vi "SubVI PhaseSpace.vi"() -> ()   [LabVIEW 2021]
uses:
  ctrOWLMarker.ctl
  ctlSeqFNs_SubVI PhaseSpace.ctl
  ctlPkgPhaseSpace.ctl
  ctlSeqFNs_SubVI ATI.ctl
  ctlTrialState.ctl
  ctlSeqFNs.ctl
  ctrSetsFlags.ctl
  ctrCommonFlags.ctl
  ctldistance2plane.ctl
  ctlRecording.ctl
  GLOBAL -MAIN.vi
  C:/Program Files/Phasespace/libowlsock.dll
panel:
  out "bias frame [R T]":dbl[][](array[numeric]) format="%#.2f"
  out "marker condition":bool[](array[boolean])
  in  "marker count":i32=14
  out "Hz":dbl(graph)
  out "save file":path
  in  "Read Cycle Time (s)":dbl=0.02 min=0.01 max=10.0 step=0.01 format="%.2f"
  out "recording?":bool
  out "markers obtained (err: <0)":u16
  out "markers":T1[](array[typedef])
  out "connected?":bool
  in  "server IP":string="192.168.1.230"
  in  "STOP":bool
  # "Parallel SubVI PhaseSpace"
  # "Acquires PhaseSpace data and Trigger signal\nSaves TDMS file."
  # "00   01  02  03   04  05   06  07  08  09   10  11   12  13"
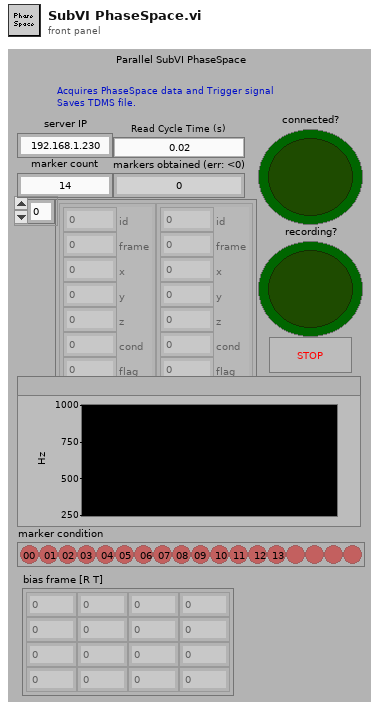
[diagram p1: front panel]
types:
  T1 = typedef "ctrOWLMarker.ctl" = cluster{"id":i32, "frame":i32, "x":sgl, "y":sgl, "z":sgl, "cond":sgl, "flag":u32}
  T2 = typedef "ctlPkgPhaseSpace.ctl" = cluster{"VIRef":refnum<vi>, "PhaseSpace":refnum<k34>, "PhaseSpace Ch names":string[], "Markers":T1[], "Markers Ch count":i32, "tick ini":i64, "ATI":refnum<queue>, "Trigger events":T3, "connected to server?":bool, "recording?":bool, "MAIN":refnum<queue>, "tick pre":i64, "Markers count":u16, "Data":dbl[][]}
  T3 = typedef "ctlTrialState.ctl" = enum16{"no events", "ready", "start", "hold", "stop", "end"}
  T4 = typedef "ctlSeqFNs_SubVI PhaseSpace.ctl" = enum16{"INITIALIZE", "IDLE", "BIAS", "READY", "SEND2MAIN", "LOG2TDMS", "TRIGGER", "END", "ERROR", "EXIT"}
  T5 = typedef "ctlSeqFNs.ctl" = enum16{"INITIALIZE MAIN", "UpdateProtocol", "UpdateBlockInfo", "UpdatePath", "INITIALIZE Sub", "IDLE", "Bias", "Ready", "RepeatTrial", "Events", "Get PS bias", "Get PhaseSpace", "Get ATI", "Finish", "End PhaseSpace", "End ATI", "ERROR", "EXIT"}
  T6 = typedef "ctlSeqFNs_SubVI ATI.ctl" = enum16{"INITIALIZE", "SET HANDLE", "IDLE", "READY", "SEND2MAIN", "CALIB Load", "BIAS", "TRIGGER", "END", "ERROR", "EXIT"}
  T7 = enum16{"ALIGN -CENTER", "ALIGN -TOP LEFT", "ALIGN -AS IS", "ALIGN -CUSTOM"}
  T8 = typedef "ctldistance2plane.ctl" = cluster{"frame":dbl[][]}
  T9 = typedef "ctlRecording.ctl" = cluster{"recording?":bool, "tdms file":refnum<k34>}
  T10 = typedef "ctrCommonFlags.ctl" = u16
  T11 = typedef "ctrSetsFlags.ctl" = u16
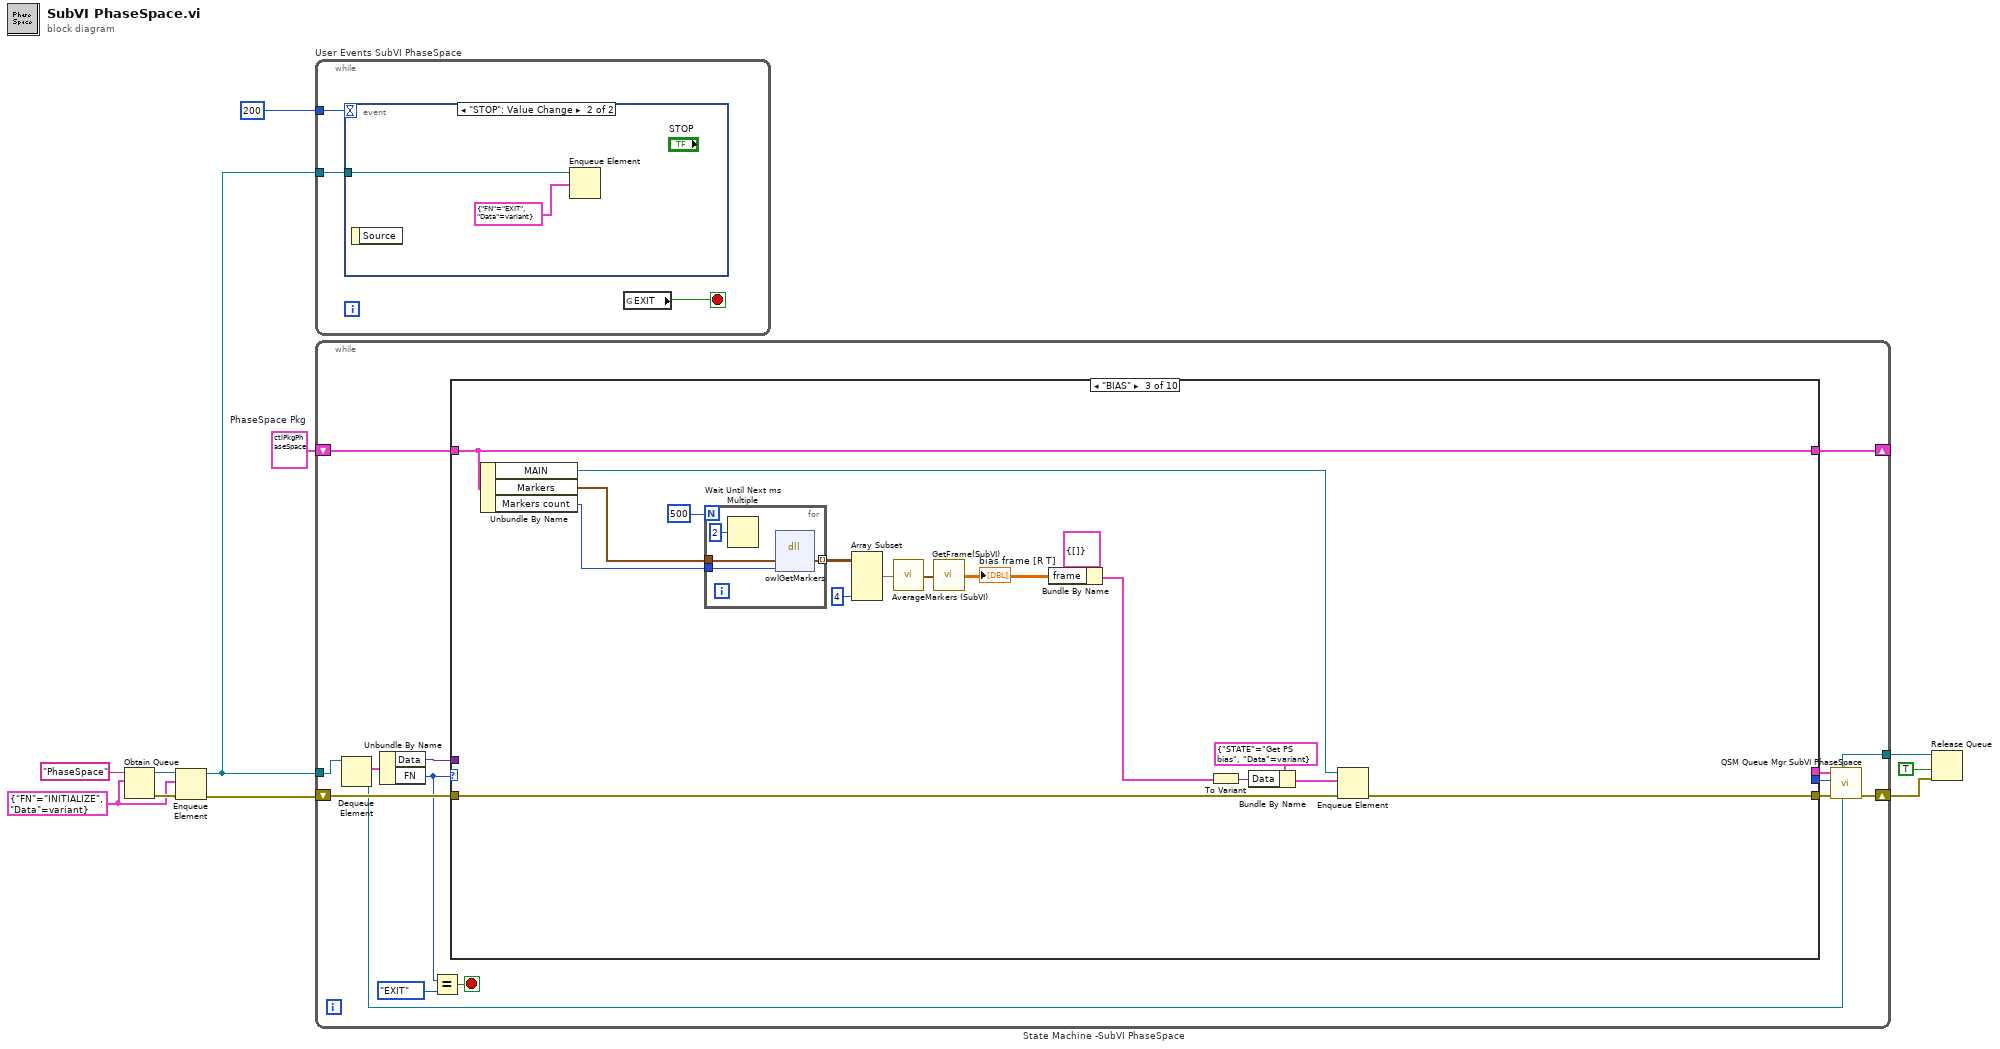
[diagram p0: block diagram]
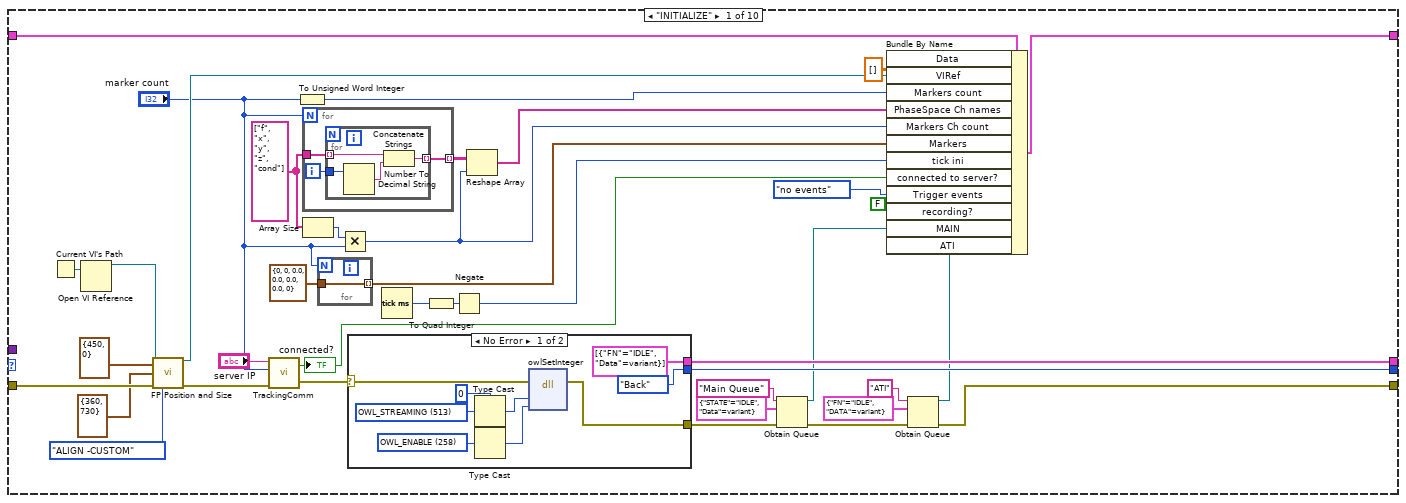
[diagram p2: hidden frame]
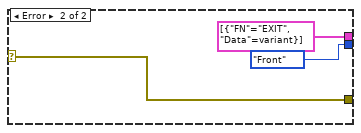
[diagram p3: hidden frame]
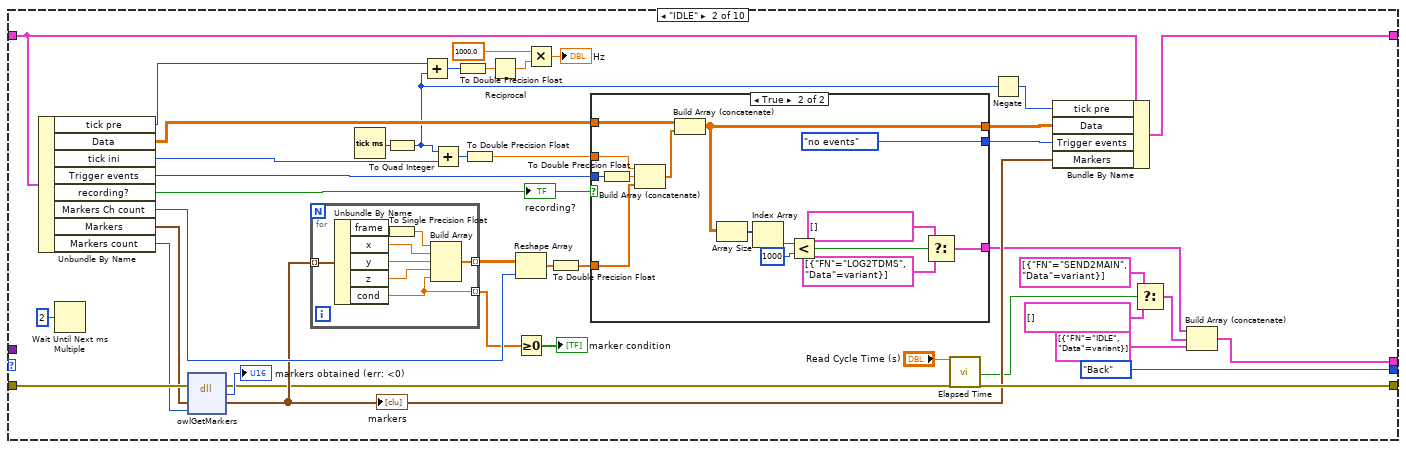
[diagram p4: hidden frame]
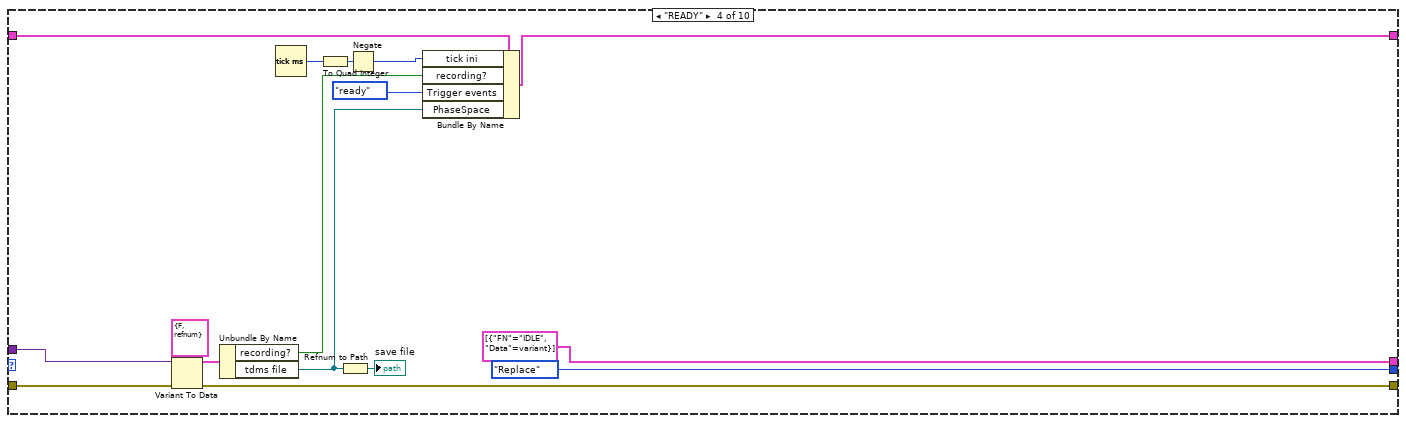
[diagram p6: hidden frame]
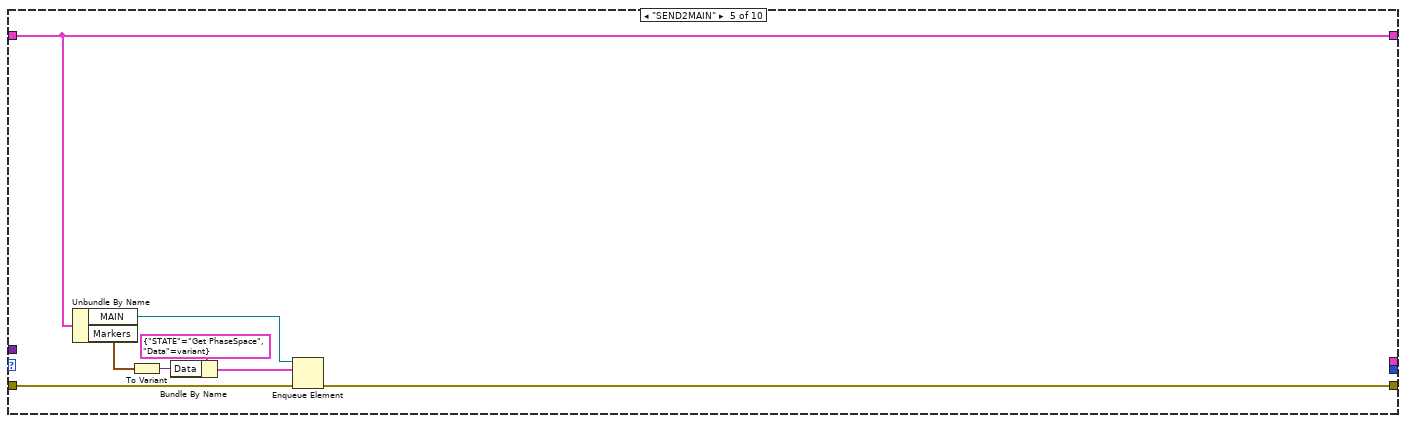
[diagram p7: hidden frame]
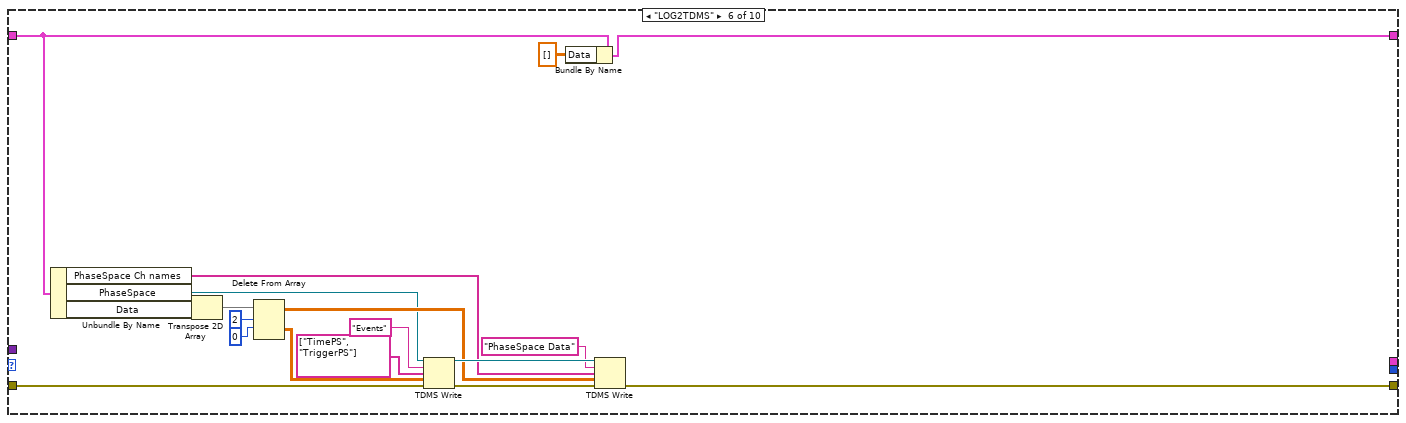
[diagram p8: hidden frame]
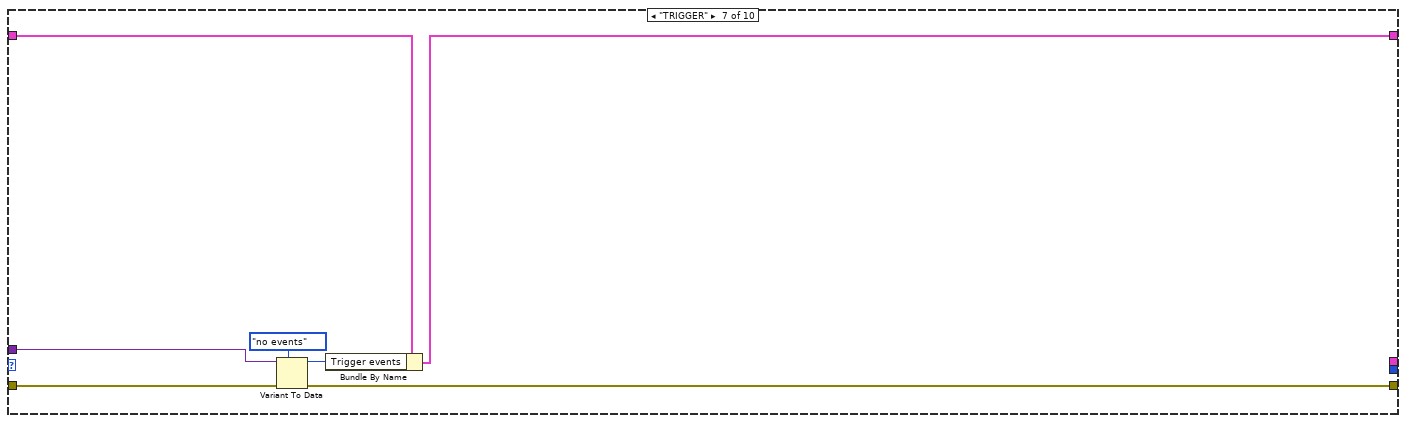
[diagram p9: hidden frame]
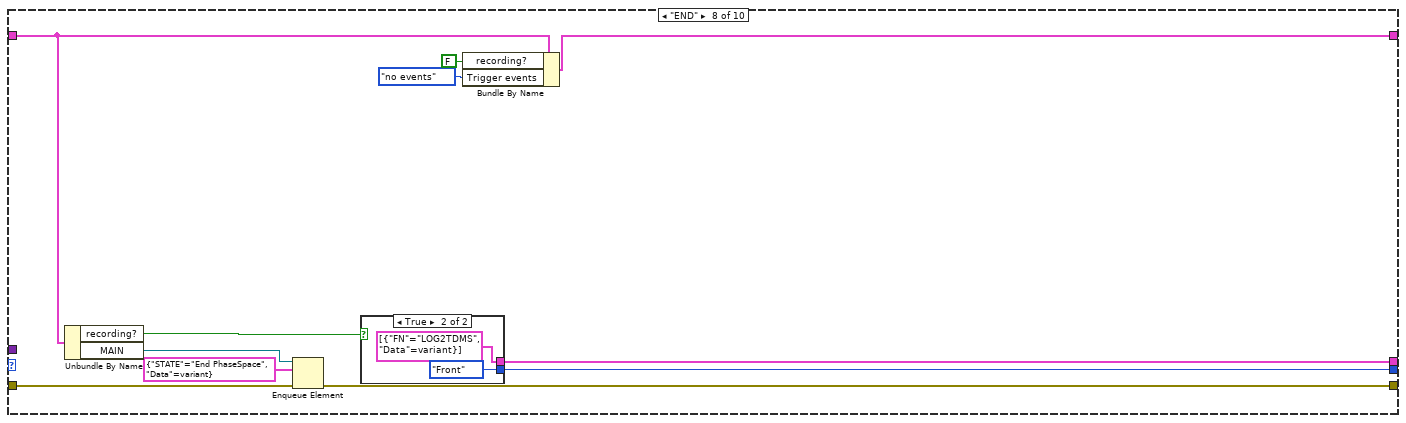
[diagram p10: hidden frame]
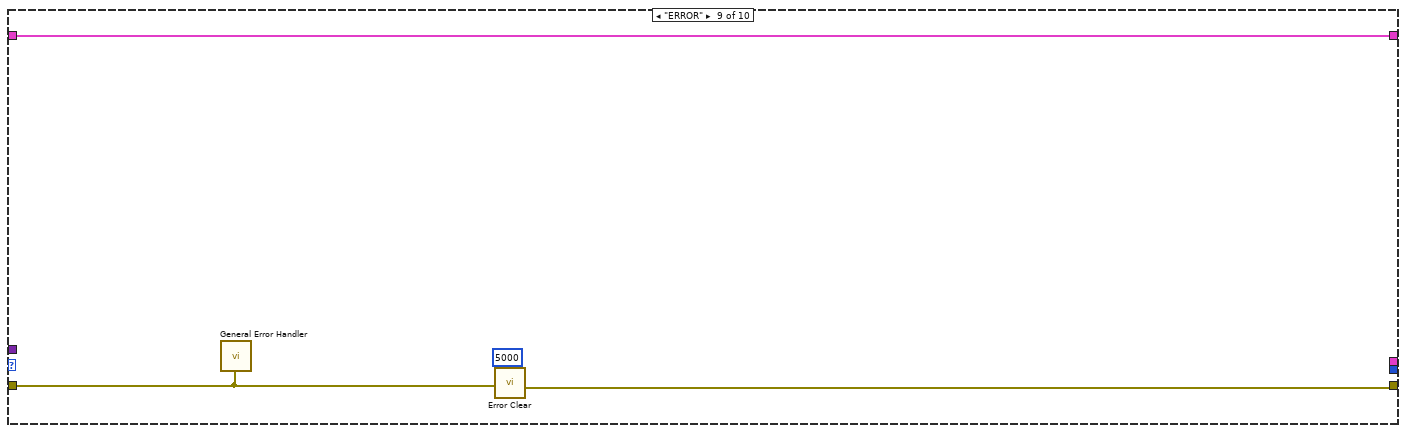
[diagram p12: hidden frame]
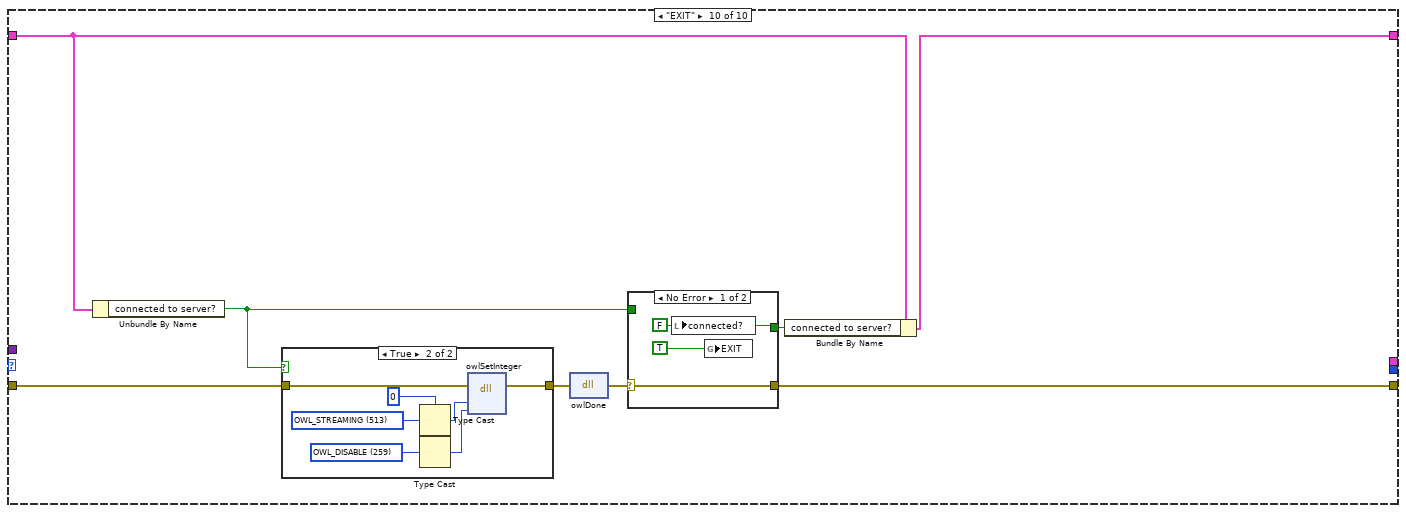
[diagram p13: hidden frame]
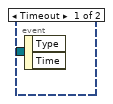
[diagram p16: hidden frame]
diagram:
  w2 = T2 {"VIRef"=refnum, "PhaseSpace"=refnum, "PhaseSpace Ch names"=[], "Markers"=[], "Markers Ch count"=0, "tick ini"=0, "ATI"=refnum, "Trigger events"=enum."no events", "connected to server?"=FALSE, "recording?"=FALSE, "MAIN"=refnum, "tick pre"=0, "Markers count"=0, "Data"=[]}  # PhaseSpace Pkg
  w6 = cluster{"FN":T4, "Data":variant} {"FN"=enum."INITIALIZE", "Data"=variant} ("cluFNData")
  n1 = Obtain Queue(name (unnamed)="PhaseSpace", element data type=w6) -> (queue out=w7:refnum<queue>, error out=w9:errorcluster)  [unwired: 3 in, 1 out]
  n2 = Enqueue Element(queue=w7, element=w6, error in (no error)=w9) -> (queue out=w3:refnum<queue>, error out=w8:errorcluster)  [unwired: 1 in, 1 out]
  n3 = while "User Events SubVI PhaseSpace" {
    tunnel: 200 -> [w14]
    tunnel: w3 -> [w12]
    stop <- w13 stop-if-true
    n4 = event shown="[1] \"STOP\": Value Change" {
      selector: _ -> [_ _]
      dyn-events: _ -> [_ _]
      timeout: w14 -> [_ _]
      tunnel: w12 -> [_ w16]
      event Timeout {
        n5 = event-data() -> ()  [unwired: 1 in, 2 out]
      }
      event "STOP": Value Change {
        n6 = event-data() -> ()  [unwired: 1 in, 1 out]
        n7 = Enqueue Element(queue=w16, element=cluster{"FN":T4, "Data":variant} {"FN"=enum."EXIT", "Data"=variant}) -> ()  [unwired: 2 in, 3 out]
      }
    }
    n8 = global read "GLOBAL -MAIN.vi" "EXIT"() -> (w13:bool)
  }
  n9 = while "State Machine -SubVI PhaseSpace" {
    shift-right: [w20] -> w1
    shift-left: w8 -> [w30]
    tunnel: w3 -> [w27]
    tunnel: [w17] -> w5
    shift-right: [w22] -> _
    shift-left: w2 -> [w23]
    stop <- w29 stop-if-true
    n10 = Dequeue Element(queue=w27) -> (queue out=w17:refnum<queue>, element=w26:cluster{"FN":T4, "Data":variant})  [unwired: 2 in, 2 out]
    n11 = Unbundle By Name(w26) -> ("Data"=w25:variant, "FN"=w24:T4)
    n12 = Equal?(x=w24, y=ctlSeqFNs_SubVI_PhaseSpace."EXIT" ("FN")) -> (x = y?=w29:bool)
    n13 = case shown="\"BIAS\"" w24 {
      tunnel: w30 -> [w67 w131 w173 w182 w201 w217 w226 w230 w240 w244]
      tunnel: [w62 w127 w172 w180 w200 w216 w225 w231 w242 w245] -> w21
      tunnel: w25 -> [_ _ _ w181 _ _ w224 _ _ _]
      tunnel: w23 -> [w49 w126 w171 w190 w199 w219 w222 w232 w243 w250]
      tunnel: [w66 w125 w171 w193 w199 w218 w223 w237 w243 w249] -> w22
      tunnel: [w44 w128 _ cluster{"FN":T4, "Data":variant}[] [{"FN"=enum."IDLE", "Data"=variant}] ("QFNs") _ _ _ w229 _ _] -> w18
      tunnel: [w43 enum16{"Back", "Front", "Replace"}."Back" ("Enum") _ enum16{"Back", "Front", "Replace"}."Replace" ("Enum") _ _ _ w228 _ _] -> w19
      frame "INITIALIZE" {
        w50 = string[] ["f", "x", "y", "z", "cond"]
        n14 = Current VI's Path() -> (path=w69:path)
        n15 = Open VI Reference(vi path=w69) -> (vi reference=w68:refnum<vi>)  [unwired: 5 in, 1 out]
        n16 = call "FP Position and Size.vi"("VIRefNum  IN"=w68, "Poistion"=cluster{"left":i16, "top":i16} {"left"=450, "top"=0}, "Size"=cluster{"right":i16, "bottom":i16} {"right"=360, "bottom"=730}, "error in (no error)"=w67, "Mode"=T7."ALIGN -CUSTOM") -> ("VIRefNum OUT"=w34:refnum<vi>, "error out"=w56:errorcluster)  [unwired: 9 in]
        n17 = call "TrackingComm.vi"("error in (no error)"=w56, "marker tally (default: 32)"="marker count", "server address"="server IP") -> ("error out"=w57:errorcluster, "connected to server?"=w41:bool)  [unwired: 1 in]
        "connected?" <- w41
        n18 = To Unsigned Word Integer(number="marker count") -> (unsigned 16bit integer=w33:u16)
        n19 = for {
          N: "marker count" -> [_]
          tunnel: w50 -> [w72]
          tunnel: [w70] -> w54 mode=indexing
          i -> [w71]
          n20 = for {
            tunnel: w72 -> [w76] mode=indexing
            tunnel: w71 -> [w75]
            tunnel: [w73] -> w70 mode=indexing
            n21 = Number To Decimal String(number=w75) -> (decimal integer string=w74:string)  [unwired: 1 in]
            n22 = Concatenate Strings(w76, w74) -> (w73:string)
          }
        }
        n23 = Array Size(array=w50) -> (size(s)=w51:i32)
        n24 = for {
          N: "marker count" -> [_]
          tunnel: T1 {"id"=0, "frame"=0, "x"=0.0, "y"=0.0, "z"=0.0, "cond"=0.0, "flag"=0} -> [w89]
          tunnel: [w89] -> w46 mode=indexing
        }
        n25 = Multiply(x=w51, y="marker count") -> (x*y=w45:i32)
        n26 = case shown="No Error" w57 {
          selector: w57 -> [w80 w88]
          tunnel: [w79 w88] -> w55
          tunnel: [cluster{"FN":T4, "Data":variant}[] [{"FN"=enum."IDLE", "Data"=variant}] ("QFNs") cluster{"FN":T4, "Data":variant}[] [{"FN"=enum."EXIT", "Data"=variant}] ("QFNs")] -> w44
          tunnel: [enum16{"Back", "Front", "Replace"}."Back" ("Enum") enum16{"Back", "Front", "Replace"}."Front" ("Enum")] -> w43
          frame No Error {
            w85 = u16 0
            w82 = T10 258 items=["OWL_CREATE"=256, "OWL_DESTROY"=257, "OWL_ENABLE"=258, "OWL_DISABLE"=259] ("Common flages")
            w81 = T11 513 items=["OWL_FREQUENCY"=512, "OWL_STREAMING"=513, "OWL_INTERPOLATION"=514, "OWL_BUTTONS"=528, "OWL_MARKERS"=529, "OWL_RIGIDS"=530, "OWL_COMMDATA"=544, "OWL_TIMESTAMP"=545, "OWL_PLANES"=672, "OWL_DETECTORS"=673, "OWL_IMAGES"=674, "OWL_TRANSFORM"=49664] ("Sets flags")
            n27 = Type Cast(type=w85, x=w81) -> (*(type *) &x=w84:u16)
            n28 = Type Cast(type=w85, x=w82) -> (*(type *) &x=w83:u16)
            n29 = dll-call lib="C:/Program Files/Phasespace/libowlsock.dll" fn="owlSetInteger"(error in=w80, "pname"=w84, "param"=w83) -> (error out=w79:errorcluster)  [unwired: 4 in, 2 out]
          }
          frame Error {
          }
        }
        n30 = Tick Count (ms)() -> (millisecond timer value=w52:u32)
        n31 = To Quad Integer(1:w52) -> (0:w53:i64)
        n32 = Negate(x=w53) -> (-x=w48:i64)
        n33 = Reshape Array(w54, w45) -> (w47:string[])
        n34 = Obtain Queue(name (unnamed)="Main Queue", element data type=cluster{"STATE":T5, "Data":variant} {"STATE"=enum."IDLE", "Data"=variant} ("element"), error in (no error)=w55) -> (queue out=w36:refnum<queue>, error out=w40:errorcluster)  [unwired: 2 in, 1 out]
        n35 = Obtain Queue(name (unnamed)="ATI", element data type=cluster{"FN":T6, "DATA":variant} {"FN"=enum."IDLE", "DATA"=variant} ("cluFNData"), error in (no error)=w40) -> (queue out=w37:refnum<queue>, error out=w62:errorcluster)  [unwired: 2 in, 1 out]
        n36 = Bundle By Name(cluster=w49, "Data"=dbl[][] [], "VIRef"=w34, "Markers count"=w33, "PhaseSpace Ch names"=w47, "Markers Ch count"=w45, "Markers"=w46, "tick ini"=w48, "connected to server?"=w41, "Trigger events"=ctlTrialState."no events", "recording?"=FALSE, "MAIN"=w36, "ATI"=w37) -> (w66:T2)
      }
      frame "IDLE" {
        n37 = Unbundle By Name(w126) -> ("tick pre"=w101:i64, "Data"=w100:dbl[][], "tick ini"=w96:i64, "Trigger events"=w93:T3, "recording?"=w129:bool, "Markers Ch count"=w112:i32, "Markers"=w124:T1[], "Markers count"=w117:u16)
        "recording?" <- w129
        n38 = Wait Until Next ms Multiple(millisecond multiple=u32 2) -> ()  [unwired: 1 out]
        n39 = dll-call lib="C:/Program Files/Phasespace/libowlsock.dll" fn="owlGetMarkers"(error in=w131, "markers"=w124, "count"=w117) -> (error out=w102:errorcluster, "return type"=→"markers obtained (err: <0)":u16, "markers"=w108:T1[])  [unwired: 3 in, 1 out]
        "markers" <- w108
        n40 = for {
          tunnel: w108 -> [w139] mode=indexing
          tunnel: [w135] -> w113 mode=indexing
          tunnel: [w132] -> w91 mode=indexing
          n41 = Unbundle By Name(w139) -> ("frame"=w134:i32, "x"=w138:sgl, "y"=w137:sgl, "z"=w136:sgl, "cond"=w132:sgl)
          n42 = To Single Precision Float(number=w134) -> (single precision float=w133:sgl)
          n43 = Build Array(w133, w138, w137, w136, w132) -> (w135:sgl[])
        }
        n44 = Tick Count (ms)() -> (millisecond timer value=w116:u32)
        n45 = To Quad Integer(1:w116) -> (0:w92:i64)
        n46 = Add(x=w101, y=w92) -> (x+y=w121:i64)
        n47 = Add(x=w92, y=w96) -> (x+y=w97:i64)
        n48 = To Double Precision Float(number=w121) -> (double precision float=w120:dbl)
        n49 = To Double Precision Float(number=w97) -> (double precision float=w95:dbl)
        n50 = Reciprocal(x=w120) -> (1/x=w122:dbl)
        n51 = Reshape Array(w113, w112) -> (w111:sgl[])
        n52 = Greater Or Equal To 0?(x=w91) -> (x >= 0?=→"marker condition":bool[])
        n53 = Multiply(x=1000.0, y=w122) -> (x*y=→"Hz":dbl)
        n54 = To Double Precision Float(number=w111) -> (double precision float=w94:dbl[])
        n55 = case shown="True" w129 {
          tunnel: w93 -> [w141 w144]
          tunnel: [w141 ctlTrialState."no events" ("Trigger events")] -> w99
          tunnel: w95 -> [_ w145]
          tunnel: w94 -> [_ w143]
          tunnel: [w140 w153] -> w98
          tunnel: w100 -> [w140 w154]
          tunnel: [_ w151] -> w107
          frame False {
          }
          frame True {
            n56 = To Double Precision Float(number=w144) -> (double precision float=w142:dbl)
            n57 = Build Array (concatenate)(w145, w142, w143) -> (w155:dbl[])
            n58 = Build Array (concatenate)(w154, w155) -> (w153:dbl[][])
            n59 = Array Size(array=w153) -> (size(s)=w152:i32[])
            n60 = Index Array(array=w152) -> (element=w148:i32)  [unwired: 1 in]
            n61 = Less?(x=w148, y=1000) -> (x < y?=w146:bool)
            n62 = Select(t=cluster{"FN":T4, "Data":variant}[] [] ("f"), s=w146, f=cluster{"FN":T4, "Data":variant}[] [{"FN"=enum."LOG2TDMS", "Data"=variant}] ("QFNs")) -> (s? t:f=w151:cluster{"FN":T4, "Data":variant}[])
          }
        }
        n63 = call "Elapsed Time"("Time Target (s)"="Read Cycle Time (s)", "error in (no error)"=w102) -> ("Time has Elapsed"=w104:bool, "error out"=w127:errorcluster)  [unwired: 10 in, 6 out]
        n64 = Negate(x=w92) -> (-x=w115:i64)
        n65 = Bundle By Name(cluster=w126, "tick pre"=w115, "Data"=w98, "Trigger events"=w99, "Markers"=w108) -> (w125:T2)
        n66 = Select(t=cluster{"FN":T4, "Data":variant}[] [{"FN"=enum."SEND2MAIN", "Data"=variant}] ("QFNs"), s=w104, f=cluster{"FN":T4, "Data":variant}[] []) -> (s? t:f=w106:cluster{"FN":T4, "Data":variant}[])
        n67 = Build Array (concatenate)(w107, w106, cluster{"FN":T4, "Data":variant}[] [{"FN"=enum."IDLE", "Data"=variant}] ("QFNs")) -> (w128:cluster{"FN":T4, "Data":variant}[])
      }
      frame "BIAS" {
        n68 = Unbundle By Name(w171) -> ("MAIN"=w165:refnum<queue>, "Markers"=w162:T1[], "Markers count"=w161:u16)
        n69 = for {
          N: 500 -> [_]
          tunnel: w162 -> [w177]
          tunnel: w161 -> [w176]
          tunnel: [w174] -> w160 mode=indexing
          n70 = Wait Until Next ms Multiple(millisecond multiple=u32 2) -> ()  [unwired: 1 out]
          n71 = dll-call lib="C:/Program Files/Phasespace/libowlsock.dll" fn="owlGetMarkers"("markers"=w177, "count"=w176) -> ("markers"=w174:T1[])  [unwired: 4 in, 3 out]
        }
        n72 = Array Subset(array=w160, length (col)=4 ("length")) -> (w159:T1[][])  [unwired: 3 in]
        n73 = call "AverageMarkers (SubVI).vi"("Markers"=w159) -> ("Avg Markers"=w158:T1[])
        n74 = call "GetFrame(SubVI).vi"("pt"=w158) -> ("frame [R T]"=w164:dbl[][])
        "bias frame [R T]" <- w164
        n75 = Bundle By Name(cluster=T8 {"frame"=[]}, "frame"=w164) -> (w166:T8)
        n76 = To Variant(anything=w166) -> (Variant=w170:variant)
        n77 = Bundle By Name(cluster=cluster{"STATE":T5, "Data":variant} {"STATE"=enum."Get PS bias", "Data"=variant} ("element"), "Data"=w170) -> (w168:cluster{"STATE":T5, "Data":variant})
        n78 = Enqueue Element(queue=w165, element=w168, error in (no error)=w173) -> (error out=w172:errorcluster)  [unwired: 1 in, 2 out]
      }
      frame "READY" {
        n79 = Variant To Data(error in=w182, type=T9 {"recording?"=FALSE, "tdms file"=refnum} ("output cluster"), Variant=w181) -> (data=w184:T9, error out=w180:errorcluster)
        n80 = Unbundle By Name(w184) -> ("recording?"=w178:bool, "tdms file"=w179:refnum<k34>)
        n81 = Tick Count (ms)() -> (millisecond timer value=w189:u32)
        n82 = To Quad Integer(1:w189) -> (0:w188:i64)
        n83 = Refnum to Path(1:w179) -> (0:→"save file":path)
        n84 = Negate(x=w188) -> (-x=w187:i64)
        n85 = Bundle By Name(cluster=w190, "tick ini"=w187, "recording?"=w178, "Trigger events"=ctlTrialState."ready", "PhaseSpace"=w179) -> (w193:T2)
      }
      frame "SEND2MAIN" {
        n86 = Unbundle By Name(w199) -> ("MAIN"=w198:refnum<queue>, "Markers"=w197:T1[])
        n87 = To Variant(anything=w197) -> (Variant=w196:variant)
        n88 = Bundle By Name(cluster=cluster{"STATE":T5, "Data":variant} {"STATE"=enum."Get PhaseSpace", "Data"=variant} ("element"), "Data"=w196) -> (w194:cluster{"STATE":T5, "Data":variant})
        n89 = Enqueue Element(queue=w198, element=w194, error in (no error)=w201) -> (error out=w200:errorcluster)  [unwired: 1 in, 2 out]
      }
      frame "LOG2TDMS" {
        n90 = Unbundle By Name(w219) -> ("PhaseSpace Ch names"=w203:string[], "PhaseSpace"=w202:refnum<k34>, "Data"=w212:dbl[][])
        n91 = Transpose 2D Array(2D array=w212) -> (transposed array=w205:dbl[][])
        n92 = Delete From Array(array=w205, length=2, index (row)=0) -> (deleted portion=w208:dbl[][], array with subset deleted=w207:dbl[][])  [unwired: 1 in]
        n93 = TDMS Write(0:w202, 5:"Events" ("group name"), 7:string[] ["TimePS", "TriggerPS"], 9:w208, 11:w217) -> (4:w215:refnum<k34>, 15:w214:errorcluster)  [unwired: 1 in, 2 out]
        n94 = Bundle By Name(cluster=w219, "Data"=dbl[][] []) -> (w218:T2)
        n95 = TDMS Write(0:w215, 5:"PhaseSpace Data" ("group name"), 7:w203, 9:w207, 11:w214) -> (15:w216:errorcluster)  [unwired: 1 in, 3 out]
      }
      frame "TRIGGER" {
        n96 = Variant To Data(error in=w226, type=ctlTrialState."no events" ("Trigger events"), Variant=w224) -> (data=w220:T3, error out=w225:errorcluster)
        n97 = Bundle By Name(cluster=w222, "Trigger events"=w220) -> (w223:T2)
      }
      frame "END" {
        n98 = Unbundle By Name(w232) -> ("recording?"=w227:bool, "MAIN"=w234:refnum<queue>)
        n99 = Enqueue Element(queue=w234, element=cluster{"STATE":T5, "Data":variant} {"STATE"=enum."End PhaseSpace", "Data"=variant}, error in (no error)=w230) -> (error out=w231:errorcluster)  [unwired: 1 in, 2 out]
        n100 = case shown="True" w227 {
          tunnel: [_ cluster{"FN":T4, "Data":variant}[] [{"FN"=enum."LOG2TDMS", "Data"=variant}] ("QFNs")] -> w229
          tunnel: [_ enum16{"Back", "Front", "Replace"}."Front" ("Enum")] -> w228
          frame False {
          }
          frame True {
          }
        }
        n101 = Bundle By Name(cluster=w232, "recording?"=FALSE, "Trigger events"=ctlTrialState."no events") -> (w237:T2)
      }
      frame "ERROR" {
        n102 = call <vilib>:"General Error Handler.vi"("error in (no error)"=w240) -> ()  [unwired: 10 in, 5 out]
        n103 = call "Error Clear.vi"("wait(ms)"=u32 5000, "error in"=w240) -> ("error in (no error)"=w242:errorcluster)  [unwired: 6 in]
      }
      frame "EXIT" {
        n104 = Unbundle By Name(w250) -> ("connected to server?"=w246:bool)
        n105 = case shown="True" w246 {
          tunnel: w244 -> [w257 w259]
          tunnel: [w257 w258] -> w251
          frame False {
          }
          frame True {
            w262 = u16 0
            w261 = T10 259 items=["OWL_CREATE"=256, "OWL_DESTROY"=257, "OWL_ENABLE"=258, "OWL_DISABLE"=259] ("Common flages")
            w260 = T11 513 items=["OWL_FREQUENCY"=512, "OWL_STREAMING"=513, "OWL_INTERPOLATION"=514, "OWL_BUTTONS"=528, "OWL_MARKERS"=529, "OWL_RIGIDS"=530, "OWL_COMMDATA"=544, "OWL_TIMESTAMP"=545, "OWL_PLANES"=672, "OWL_DETECTORS"=673, "OWL_IMAGES"=674, "OWL_TRANSFORM"=49664] ("Sets flags")
            n106 = Type Cast(type=w262, x=w260) -> (*(type *) &x=w263:u16)
            n107 = Type Cast(type=w262, x=w261) -> (*(type *) &x=w264:u16)
            n108 = dll-call lib="C:/Program Files/Phasespace/libowlsock.dll" fn="owlSetInteger"(error in=w259, "pname"=w263, "param"=w264) -> (error out=w258:errorcluster)  [unwired: 4 in, 2 out]
          }
        }
        n109 = dll-call lib="C:/Program Files/Phasespace/libowlsock.dll" fn="owlDone"(error in=w251) -> (error out=w248:errorcluster)  [unwired: 2 in, 2 out]
        n110 = case shown="No Error" w248 {
          selector: w248 -> [w252 w255]
          tunnel: [w254 w256] -> w247
          tunnel: w246 -> [_ w256]
          tunnel: [w252 w255] -> w245
          frame No Error {
            w254 = FALSE ("connected to server?")
            n111 = local write "connected?"(w254) -> ()
            n112 = global write "GLOBAL -MAIN.vi" "EXIT"(TRUE ("EXIT")) -> ()
          }
          frame Error {
          }
        }
        n113 = Bundle By Name(cluster=w250, "connected to server?"=w247) -> (w249:T2)
      }
    }
    n114 = call "QSM Queue Mgr SubVI PhaseSpace.vi"("QRef"=w17, "Error IN"=w21, "FNs"=w19, "QSTATES"=w18) -> ("Error OUT"=w20:errorcluster)  [unwired: 4 in]
  }
  n115 = Release Queue(queue=w5, force destroy? (F)=TRUE, error in (no error)=w1) -> ()  [unwired: 3 out]
